vi "Refresh SRs.vi"(8 "error in (no error)":errorcluster, 11 "Data Loop Data in":T1) -> (0 "error out":errorcluster, 3 "Data Loop Data out":T1)   [LabVIEW 2018]
uses:
  Type Defs/Data Loop Data.ctl
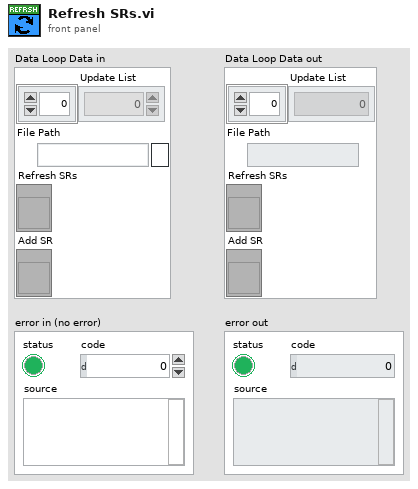
[diagram p1: front panel]
types:
  T1 = typedef "Data Loop Data.ctl" = cluster{"Update List":i32[], "File Path":path, "Refresh SRs":refnum<vi>, "Add SR":refnum<vi>}
  T2 = typedef "SR Cluster.ctl" = cluster{"Color":u32, "SR Number":i32, "SR Status":T3, "Name":string, "Summary":string, "Last Updated":timestamp, "SR Type":string, "Service Level":string, "Days Open":dbl, "Creation Date":timestamp}
  T3 = typedef "SR Status.ctl" = enum16{"Caller Abandoned", "Created in Error", "Expired", "Forum Resolved AE", "Forum Resolved Customer", "IN WORK", "IN WORK Collab with AES", "IN WORK Collab with PSE", "IN WORK Collab with SE", "IN WORK Customer Added Note", "IN WORK Escalation", "IN WORK Wait on Customer", "Open", "Potentially Resolved", "Presumed Resolved", "RMA Approved for Return", "Resolved", "Passed Off"}
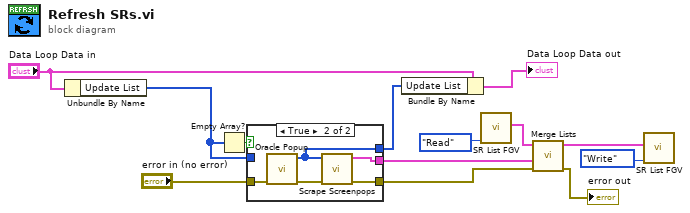
[diagram p0: block diagram]
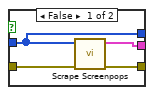
[diagram p2: hidden frame]
diagram:
  n1 = Unbundle By Name("Data Loop Data in") -> ("Update List"=w1:i32[])
  n2 = Empty Array?(array=w1) -> (empty?=w4:bool)
  n3 = case shown="True" w4 {
    tunnel: w1 -> [w14 _]
    tunnel: "error in (no error)" -> [w16 w22]
    tunnel: [w17 w20] -> w11
    tunnel: [w15 w19] -> w8
    tunnel: [w14 w21] -> w6
    frame False {
      n4 = call "Scrape Screenpops.vi"("error in"=w16, "SR number list in"=w14) -> ("error out"=w15:errorcluster, "sr clusters out"=w17:T2[])  [unwired: 8 in]
    }
    frame True {
      n5 = call "Oracle Popup.vi"("error in"=w22) -> ("error out"=w18:errorcluster, "SR number list out"=w21:i32[])  [unwired: 9 in]
      n6 = call "Scrape Screenpops.vi"("error in"=w18, "SR number list in"=w21) -> ("error out"=w19:errorcluster, "sr clusters out"=w20:T2[])  [unwired: 8 in]
    }
  }
  n7 = Bundle By Name(cluster="Data Loop Data in", "Update List"=w6) -> (→"Data Loop Data out":T1)
  n8 = call "SR List FGV.vi"("Operation"=enum16{"Initialize", "Write", "Read", "Clear"}."Read") -> ("list out"=w12:T2[])  [unwired: 9 in, 1 out]
  n9 = call "Merge Lists.vi"("error in"=w8, "new list in"=w11, "list in"=w12) -> ("error out"=→"error out":errorcluster, "list out"=w10:T2[])  [unwired: 7 in]
  n10 = call "SR List FGV.vi"("Operation"=enum16{"Initialize", "Write", "Read", "Clear"}."Write", "list in"=w10) -> ()  [unwired: 8 in, 2 out]
